vi "Read Stop Event Registration Refnum.vi"(11 "Input Device in":refnum<class "Input Device.lvclass">) -> (2 "Stop Event Registration Refnum out":refnum<event-registration>)   [LabVIEW 2024, in "Input Device.lvclass"]
doc: "MIT Licence\nCopyright (c) 2024 David Grollier"
uses:
  Input Device.lvclass
  Input Device.lvclass/Input Device.ctl
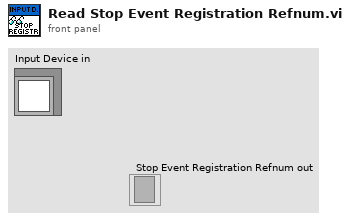
[diagram p1: front panel]
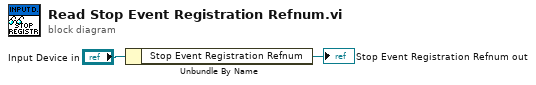
[diagram p0: block diagram]
diagram:
  n1 = Unbundle By Name("Input Device in") -> ("Stop Event Registration Refnum"=→"Stop Event Registration Refnum out":refnum<event-registration>)
